vi "Menu 2.vi"() -> ()   [LabVIEW 2015]
panel:
  in  "stop":bool
  in  "Change menu":bool
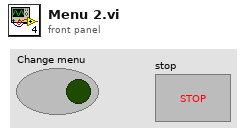
[diagram p1: front panel]
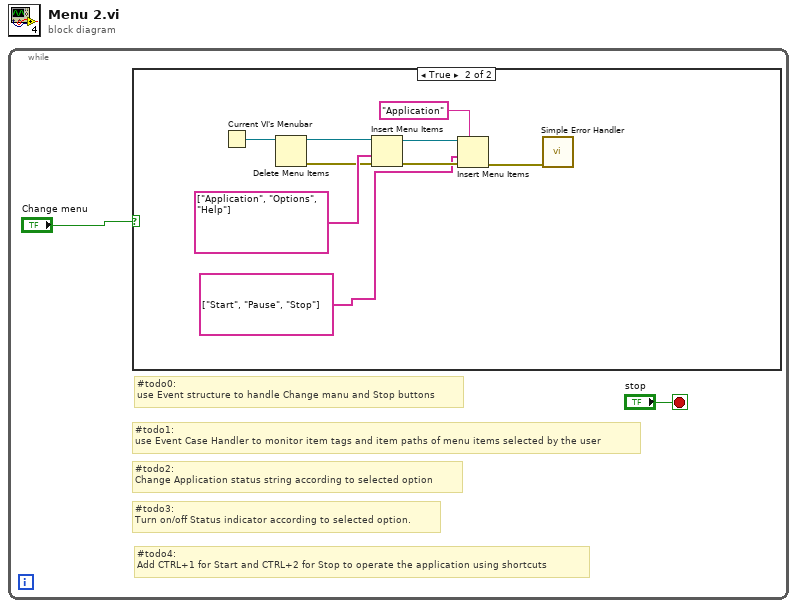
[diagram p0: block diagram]
diagram:
  n1 = while {
    stop <- "stop" stop-if-true
    # "#todo4:\nAdd CTRL+1 for Start and CTRL+2 for Stop to operate the application using shortcuts"
    # "#todo3:\nTurn on/off Status indicator according to selected option."
    # "#todo2:\nChange Application status string according to selected option"
    # "#todo1:\nuse Event Case Handler to monitor item tags and item paths of menu items selected by the user"
    # "#todo0:\nuse Event structure to handle Change manu and Stop buttons"
    n2 = case shown="True" "Change menu" {
      frame False {
      }
      frame True {
        n3 = Current VI's Menubar() -> (w9:refnum<k9>)
        n4 = Delete Menu Items(9:w9) -> (0:w8:errorcluster, 3:w10:refnum<k9>)  [unwired: 3 in]
        n5 = Insert Menu Items(6:w8, 7:string[] ["Application", "Options", "Help"] ("L10n_item tags 1"), 9:w10) -> (0:w7:errorcluster, 3:w3:refnum<k9>)  [unwired: 3 in, 1 out]
        n6 = Insert Menu Items(5:"Application" ("menu tag"), 6:w7, 7:string[] ["Start", "Pause", "Stop"] ("L10n_item tags 1"), 9:w3) -> (0:w6:errorcluster)  [unwired: 2 in, 2 out]
        n7 = call <vilib>:"Simple Error Handler.vi"("error in (no error)"=w6) -> ()  [unwired: 4 in, 5 out]
      }
    }
  }
